vi "SimpleFunc2.vi"(8 "Error In":errorcluster, 11 "cyclesCnt":i32=42) -> (0 "Error Out":errorcluster)   [LabVIEW 2014]
uses:
  C_Library/C Basic Lib.lvlib
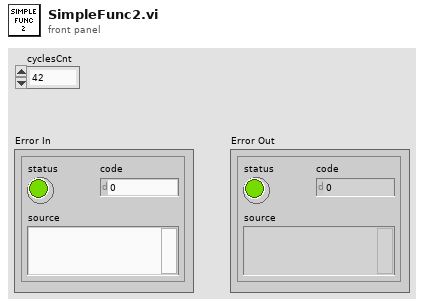
[diagram p1: front panel]
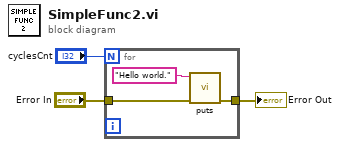
[diagram p0: block diagram]
diagram:
  n1 = for {
    N: "cyclesCnt" -> [_]
    tunnel: "Error In" -> [w6]
    tunnel: [w5] -> w1
    n2 = call "puts.vi"("error in"=w6, "String in"="Hello world.") -> ("error out"=w5:errorcluster)  [unwired: 9 in]
  }
  "Error Out" <- w1
